vi "ComputeSteeringAngle.vi"(8 "error (in)":errorcluster, 9 "Current GPS Data":T1, 10 "Previous GPS Data":T1, 11 "Waypoint Array":cluster{"Latitude":dbl, "Longitude":dbl}[](array[cluster])) -> (0 "error (out)":errorcluster, 1 "Steering Angle":dbl, 2 "Bearing to Waypoint (deg)":dbl, 3 "Current Bearing (deg)":dbl, 4 "Bearing Diff. (deg)":dbl)   [LabVIEW 2015]
doc: "Computes the steering angle needed to reach the current waypoint based on the current heading and the heading to the destination."
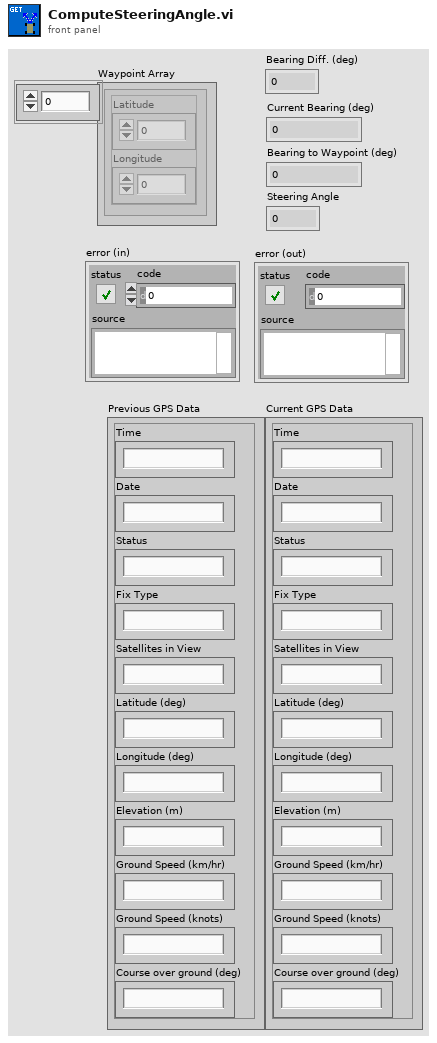
[diagram p1: front panel]
types:
  T1 = cluster{"Time":string, "Date":string, "Status":string, "Fix Type":string, "Satellites in View":string, "Latitude (deg)":string, "Longitude (deg)":string, "Elevation (m)":string, "Ground Speed (km/hr)":string, "Ground Speed (knots)":string, "Course over ground (deg)":string}
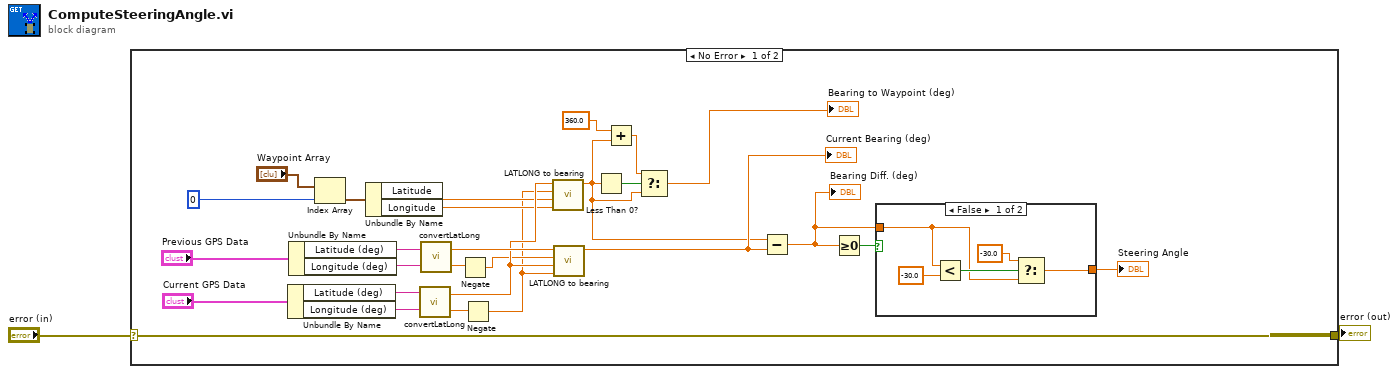
[diagram p0: block diagram]
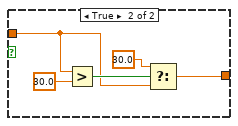
[diagram p2: hidden frame]
diagram:
  n1 = case shown="No Error" "error (in)" {
    selector: "error (in)" -> [w13 w40]
    tunnel: [w13 w40] -> w1
    frame No Error {
      n2 = Unbundle By Name("Current GPS Data") -> ("Latitude (deg)"=w25:string, "Longitude (deg)"=w24:string)
      n3 = Unbundle By Name("Previous GPS Data") -> ("Latitude (deg)"=w28:string, "Longitude (deg)"=w27:string)
      n4 = Index Array(array="Waypoint Array", index=0) -> (element=w20:cluster{"Latitude":dbl, "Longitude":dbl})
      n5 = Unbundle By Name(w20) -> ("Latitude"=w18:dbl, "Longitude"=w17:dbl)
      n6 = call "convertLatLong.vi"("Longitude (deg)"=w24, "Latitude (deg)"=w25) -> ("Longitude (deg)"=w9:dbl, "Latitude (deg)"=w19:dbl)
      n7 = call "convertLatLong.vi"("Longitude (deg)"=w27, "Latitude (deg)"=w28) -> ("Longitude (deg)"=w12:dbl, "Latitude (deg)"=w23:dbl)
      n8 = Negate(x=w12) -> (-x=w11:dbl)
      n9 = Negate(x=w9) -> (-x=w10:dbl)
      n10 = call "LATLONG to bearing.vi"("LONG2"=w17, "LAT2"=w18, "LONG1"=w10, "LAT1"=w19) -> ("Bearing (deg)"=w4:dbl)  [unwired: 5 in, 2 out]
      n11 = call "LATLONG to bearing.vi"("LONG2"=w10, "LAT2"=w19, "LONG1"=w11, "LAT1"=w23) -> ("Bearing (deg)"=w8:dbl)  [unwired: 5 in, 2 out]
      "Current Bearing (deg)" <- w8
      n12 = Less Than 0?(x=w4) -> (x < 0?=w7:bool)
      n13 = Add(x=360.0, y=w4) -> (x+y=w5:dbl)
      n14 = Select(t=w5, s=w7, f=w4) -> (s? t:f=→"Bearing to Waypoint (deg)":dbl)
      n15 = Subtract(x=w4, y=w8) -> (x-y=w15:dbl)
      "Bearing Diff. (deg)" <- w15
      n16 = Greater Or Equal To 0?(x=w15) -> (x >= 0?=w16:bool)
      n17 = case shown="False" w16 {
        tunnel: w15 -> [w31 w35]
        tunnel: [w30 w36] -> w14
        frame False {
          n18 = Less?(x=w31, y=-30.0) -> (x < y?=w34:bool)
          n19 = Select(t=-30.0, s=w34, f=w31) -> (s? t:f=w30:dbl)
        }
        frame True {
          n20 = Greater?(x=w35, y=30.0) -> (0:w39:bool)
          n21 = Select(t=30.0, s=w39, f=w35) -> (s? t:f=w36:dbl)
        }
      }
      "Steering Angle" <- w14
    }
    frame Error {
    }
  }
  "error (out)" <- w1
